vi "sub_ofdm_subcarrier_allocator.vi"(8 "fft size":i32=256, 9 "pilot symbol":cdb[](array[numeric]), 11 "message symbol":cdb[](array[numeric])) -> (3 "OFDM symbol":cdb[](array[numeric]))   [LabVIEW 2014]
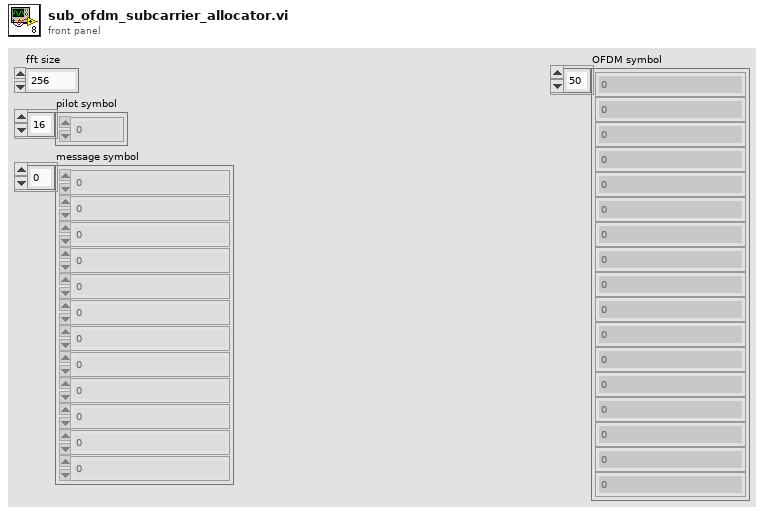
[diagram p1: front panel]
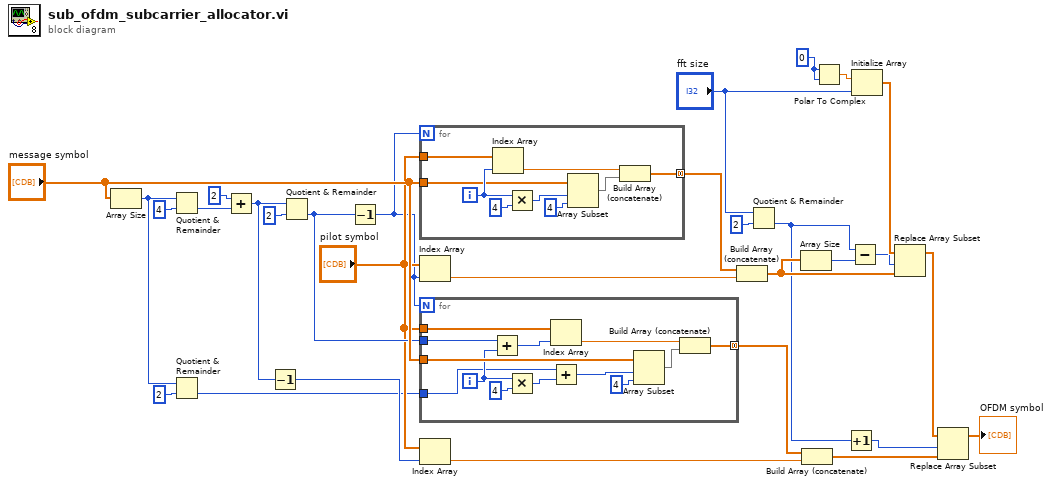
[diagram p0: block diagram]
diagram:
  w29 = 0
  n1 = Array Size(array="message symbol") -> (size(s)=w5:i32)
  n2 = Quotient & Remainder(x=w5, y=4) -> (floor(x/y)=w8:i32)  [unwired: 1 out]
  n3 = Quotient & Remainder(x=w5, y=2) -> (floor(x/y)=w3:i32)  [unwired: 1 out]
  n4 = Add(x=2, y=w8) -> (x+y=w6:i32)
  n5 = Decrement(x=w6) -> (x-1=w23:i32)
  n6 = Quotient & Remainder(x=w6, y=2) -> (floor(x/y)=w24:i32)  [unwired: 1 out]
  n7 = Decrement(x=w24) -> (x-1=w10:i32)
  n8 = for {
    N: w10 -> [_]
    tunnel: "message symbol" -> [w34]
    tunnel: "pilot symbol" -> [w39]
    tunnel: [w31] -> w27 mode=concatenating
    i -> [w37]
    n9 = Index Array(array=w39, index=w37) -> (element=w33:cdb)
    n10 = Multiply(x=w37, y=4) -> (x*y=w35:i32)
    n11 = Array Subset(array=w34, index=w35, length=4) -> (w32:cdb[])
    n12 = Build Array (concatenate)(w33, w32) -> (w31:cdb[])
  }
  n13 = Index Array(array="pilot symbol", index=w10) -> (element=w26:cdb)
  n14 = for {
    N: w10 -> [_]
    tunnel: "message symbol" -> [w49]
    tunnel: "pilot symbol" -> [w52]
    tunnel: [w46] -> w20 mode=concatenating
    tunnel: w24 -> [w42]
    tunnel: w3 -> [w40]
    i -> [w44]
    n15 = Add(x=w42, y=w44) -> (x+y=w45:i32)
    n16 = Multiply(x=w44, y=4) -> (x*y=w43:i32)
    n17 = Index Array(array=w52, index=w45) -> (element=w48:cdb)
    n18 = Add(x=w40, y=w43) -> (x+y=w41:i32)
    n19 = Array Subset(array=w49, index=w41, length=4) -> (w47:cdb[])
    n20 = Build Array (concatenate)(w48, w47) -> (w46:cdb[])
  }
  n21 = Index Array(array="pilot symbol", index=w23) -> (element=w21:cdb)
  n22 = Build Array (concatenate)(w27, w26) -> (w14:cdb[])
  n23 = Quotient & Remainder(x="fft size", y=2) -> (floor(x/y)=w2:i32)  [unwired: 1 out]
  n24 = Array Size(array=w14) -> (size(s)=w17:i32)
  n25 = Build Array (concatenate)(w20, w21) -> (w13:cdb[])
  n26 = Polar To Complex(1:w29, 2:w29) -> (0:w30:cdb)
  n27 = Increment(x=w2) -> (x+1=w1:i32)
  n28 = Subtract(x=w2, y=w17) -> (x-y=w15:i32)
  n29 = Initialize Array(w30, "fft size") -> (w16:cdb[])
  n30 = Replace Array Subset(array=w16, new element=w14, index=w15) -> (w12:cdb[])
  n31 = Replace Array Subset(array=w12, new element=w13, index=w1) -> (→"OFDM symbol":cdb[])
